vi "draw.vi"(0 "reference":refnum<class "FinalStateNode.lvclass">, 1 "graphics":refnum<class "Graphics.lvclass">, 5 "error in (no error)":errorcluster) -> (14 "reference out":refnum<class "FinalStateNode.lvclass">, 19 "error out":errorcluster)   [LabVIEW 2014, in "FinalStateNode.lvclass"]
doc: "public void draw(Graphics2D g2, Point2D p, Point2D q)"
uses:
  <resource>/Framework/Providers/Open_GDS/UML/FinalStateNode_class/FinalStateNode.lvclass
  <resource>/Framework/Providers/Open_GDS/UML/Graphics_class/Graphics.lvclass
  <resource>/Framework/Providers/Open_GDS/UML/MultiLineString_class/MultiLineString.lvclass
panel:
  in  "Case Constant\n(See Context Help)":bool
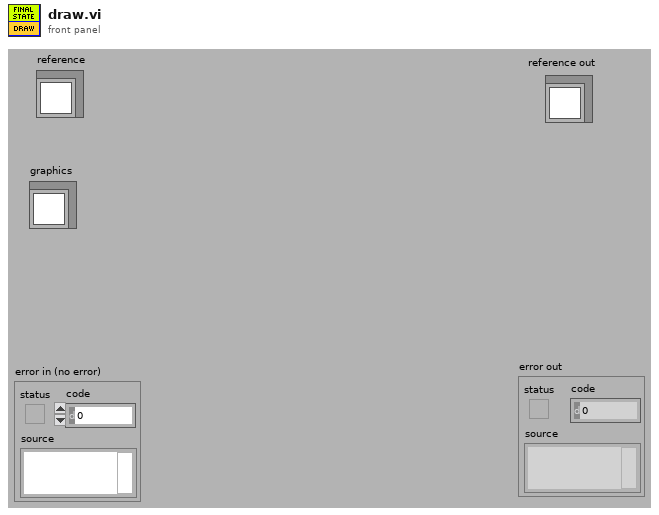
[diagram p1: front panel]
types:
  T1 = typedef "FinalStateNode.lvclass/ObjectAttributes.ctl" = cluster{"Base class":T2, "name":refnum<class "MultiLineString.lvclass">, "DEFAULT_WIDTH":i32, "DEFAULT_HEIGHT":i32}
  T2 = typedef "RectangularNode.lvclass/ObjectAttributes.ctl" = cluster{"Base class":T3, "bounds":T4}
  T3 = typedef "AbstractNode.lvclass/ObjectAttributes.ctl" = cluster{"parent":refnum<class "AbstractNode.lvclass">, "children":refnum<class "AbstractNode.lvclass">[], "Hidden":bool}
  T4 = typedef "Rectangle Rectangle2D.ctl" = cluster{"x":dbl, "y":dbl, "width":dbl, "height":dbl}
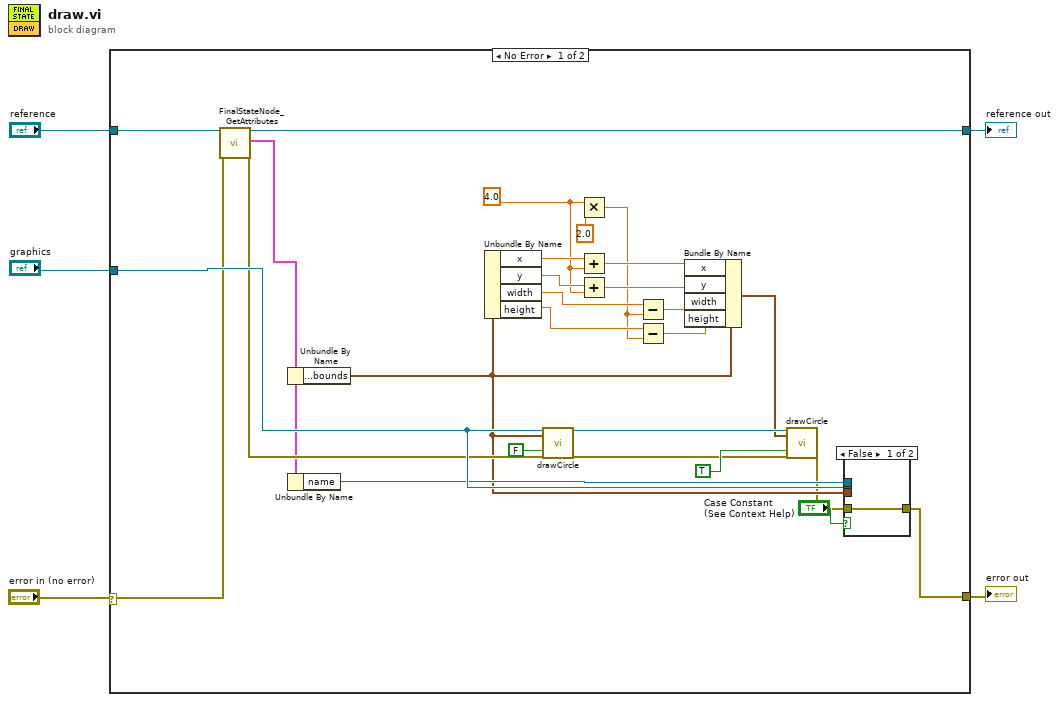
[diagram p0: block diagram]
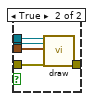
[diagram p2: hidden frame]
diagram:
  n1 = case shown="No Error" "error in (no error)" {
    selector: "error in (no error)" -> [w25 w39]
    tunnel: "reference" -> [w32 w40]
    tunnel: [w31 w39] -> w4
    tunnel: [w30 w40] -> w3
    tunnel: "graphics" -> [w29 _]
    frame No Error {
      w15 = 4.0
      n2 = call <resource>:"FinalStateNode_GetAttributes.vi"("reference in"=w32, "error in (no error)"=w25) -> ("reference out"=w30:refnum<class "FinalStateNode.lvclass">, "Attributes"=w26:T1, "error out"=w27:errorcluster)  [unwired: 15 out]
      n3 = Unbundle By Name(w26) -> ("Base class.bounds"=w14:T4)
      n4 = Unbundle By Name(w26) -> ("name"=w28:refnum<class "MultiLineString.lvclass">)
      n5 = Unbundle By Name(w14) -> ("x"=w20:dbl, "y"=w19:dbl, "width"=w18:dbl, "height"=w17:dbl)
      n6 = call-dynamic "drawCircle.vi"("reference"=w29, "rectangle"=w14, "fill?(F)"=FALSE, "error in (no error)"=w27) -> ("reference out"=w22:refnum<class "Graphics.lvclass">, "error out"=w7:errorcluster)  [unwired: 14 in]
      n7 = Multiply(x=w15, y=2.0) -> (x*y=w9:dbl)
      n8 = Add(x=w20, y=w15) -> (x+y=w13:dbl)
      n9 = Add(x=w19, y=w15) -> (x+y=w12:dbl)
      n10 = Subtract(x=w18, y=w9) -> (x-y=w11:dbl)
      n11 = Subtract(x=w17, y=w9) -> (x-y=w10:dbl)
      n12 = Bundle By Name(cluster=w14, "x"=w13, "y"=w12, "width"=w11, "height"=w10) -> (w8:T4)
      n13 = call-dynamic "drawCircle.vi"("reference"=w22, "rectangle"=w8, "fill?(F)"=TRUE, "error in (no error)"=w7) -> ("error out"=w6:errorcluster)  [unwired: 14 in, 1 out]
      n14 = case shown="False" "Case Constant\n(See Context Help)" {
        tunnel: [w33 w38] -> w31
        tunnel: w29 -> [_ w37]
        tunnel: w28 -> [_ w36]
        tunnel: w6 -> [w33 w35]
        tunnel: w14 -> [_ w34]
        frame False {
        }
        frame True {
          n15 = call-dynamic "draw.vi"("reference"=w36, "graphics"=w37, "bounds"=w34, "error in (no error)"=w35) -> ("error out"=w38:errorcluster)  [unwired: 14 in, 1 out]
        }
      }
    }
    frame Error {
    }
  }
  "reference out" <- w3
  "error out" <- w4
